vi "ThreeIncoming.vi"() -> ()   [LabVIEW 2013]
uses:
  <vilib>/rvi/Emulation/niFpgaSctlEmulationGetInTimedLoop.vi
  <vilib>/rvi/Emulation/niFpgaEmulationReportErrorSimple.vi
  <vilib>/rvi/Emulation/niFpgaGetClockAttributes.vi
  <vilib>/rvi/interface/RandomDataEmulation/nirviRandomDataFPGAFIFO.vi
  <vilib>/rvi/interface/RandomDataEmulation/niFpgaRandomDataHandleErrors.vi
  <vilib>/rvi/Emulation/niFpgaCriticalErrorInLSC.vi
  <vilib>/rvi/DataTransferAndStorage/Container/XNode/niFpgaContainer.xnode
  <vilib>/rvi/interface/RandomDataEmulation/nirviRandomDataFpgaReadWriteTemplate.vi
panel:
  out "Boolean 2":bool=TRUE
  out "Fast timeout":bool
  out "Med timeout":bool
  out "Slow timeout":bool
  in  "I16":i16
  in  "I8":i8
  in  "I64":i64
  in  "I32":i32
  in  "U16":u16
  in  "U8":u8
  in  "U64":u64
  in  "U32":u32
  in  "SGL":sgl
  in  "Boolean":bool
  out "I16 out":i16
  out "I8 out":i8
  out "I64 out":i64
  out "I32 out":i32
  out "U16 out":u16
  out "U8 out":u8
  out "U64 out":u64
  out "U32 out":u32
  out "SGL out":sgl
  out "Boolean out":bool
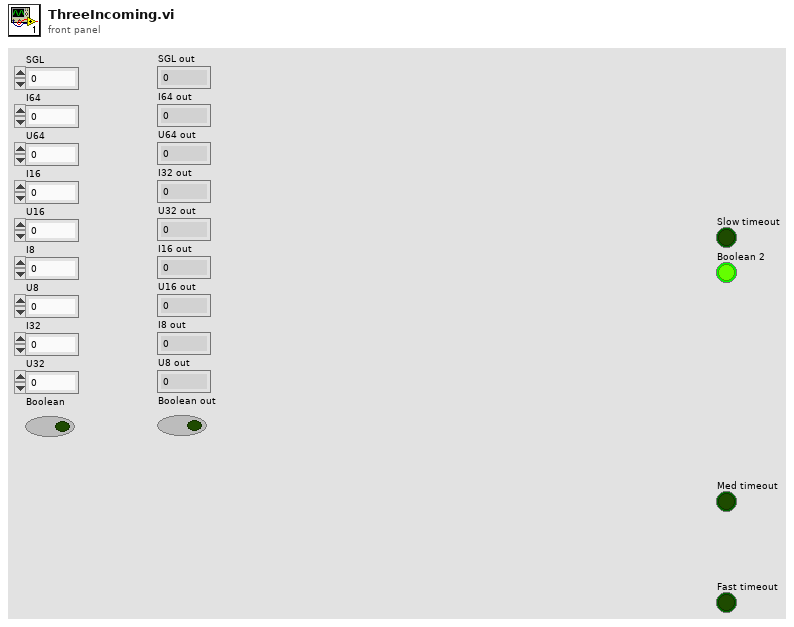
[diagram p1: front panel]
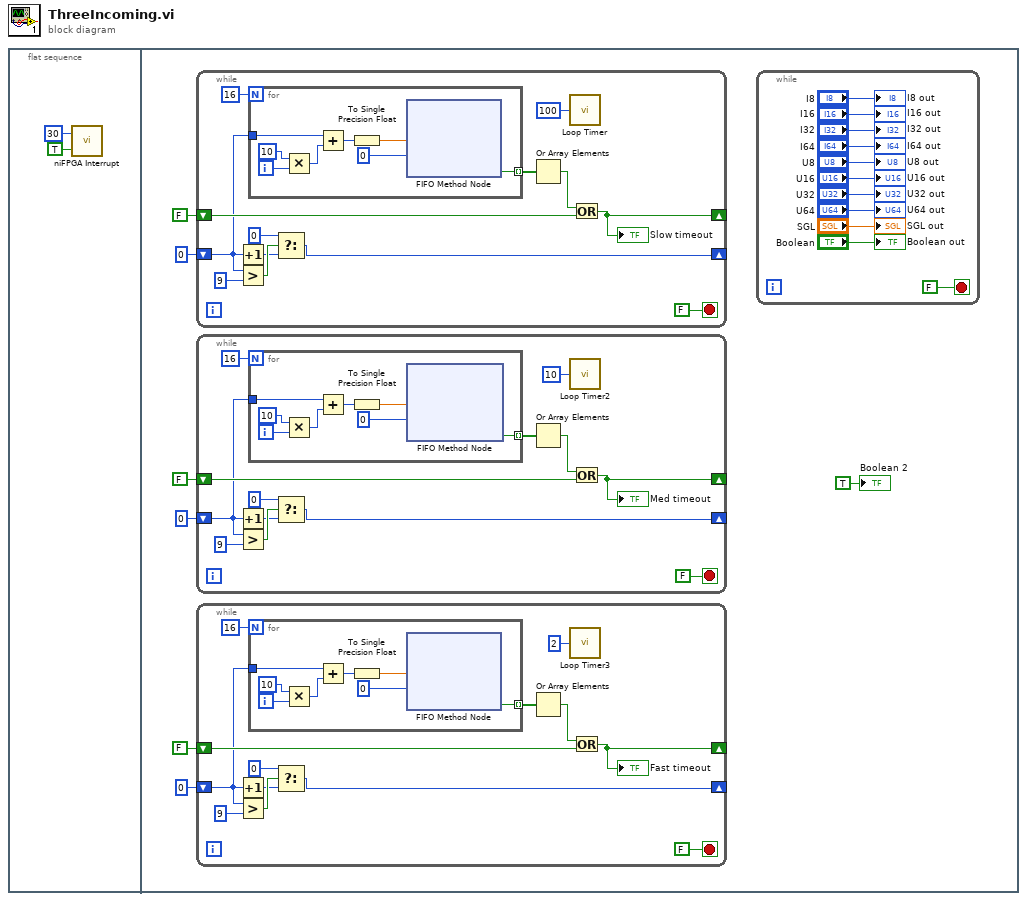
[diagram p0: block diagram]
diagram:
  n1 = flat-sequence {
    frame #0 {
      n2 = call <vilib>:"niFPGA Interrupt.vi"("Wait Until Cleared (F)"=TRUE, "IRQ Number (0)"=u8 30) -> ()  [unwired: 1 in]
    }
    frame #1 {
      n3 = while {
        shift-right: [w59] -> _
        shift-left: 0 ("t") -> [w52]
        shift-right: [w53] -> _
        shift-left: FALSE -> [w54]
        stop <- FALSE stop-if-true
        n4 = Increment(x=w52) -> (x+1=w57:i32)
        n5 = Greater?(x=w52, y=9) -> (0:w63:bool)
        n6 = for {
          N: 16 -> [_]
          tunnel: w52 -> [w72]
          tunnel: [w65] -> w56 mode=indexing
          i -> [w71]
          n7 = Multiply(x=10, y=w71) -> (x*y=w69:i32)
          n8 = Add(x=w72, y=w69) -> (x+y=w68:i32)
          n9 = To Single Precision Float(number=w68) -> (single precision float=w67:sgl)
          n10 = xnode ("FIFO Method Node")("Element"=w67, "Timeout"=0) -> ("Timed Out?"=w65:bool)  [unwired: 1 in, 1 out]
        }
        n11 = Select(t=0, s=w63, f=w57) -> (s? t:f=w59:i32)
        n12 = Or Array Elements(Boolean array=w56) -> (logical OR=w55:bool)
        n13 = call "Loop Timer"("Count(uSec)"=u32 100) -> ()  [unwired: 1 out]
        n14 = Or(x=w55, y=w54) -> (x .or. y?=w53:bool)
        "Slow timeout" <- w53
      }
      n15 = while {
        shift-right: [w38] -> _
        shift-left: 0 ("t") -> [w31]
        shift-right: [w32] -> _
        shift-left: FALSE -> [w33]
        stop <- FALSE stop-if-true
        n16 = Increment(x=w31) -> (x+1=w36:i32)
        n17 = Greater?(x=w31, y=9) -> (0:w42:bool)
        n18 = for {
          N: 16 -> [_]
          tunnel: w31 -> [w51]
          tunnel: [w44] -> w35 mode=indexing
          i -> [w50]
          n19 = Multiply(x=10, y=w50) -> (x*y=w48:i32)
          n20 = Add(x=w51, y=w48) -> (x+y=w47:i32)
          n21 = To Single Precision Float(number=w47) -> (single precision float=w46:sgl)
          n22 = xnode ("FIFO Method Node")("Element"=w46, "Timeout"=0) -> ("Timed Out?"=w44:bool)  [unwired: 1 in, 1 out]
        }
        n23 = Select(t=0, s=w42, f=w36) -> (s? t:f=w38:i32)
        n24 = Or Array Elements(Boolean array=w35) -> (logical OR=w34:bool)
        n25 = call "Loop Timer2"("Count(uSec)"=u32 10) -> ()  [unwired: 1 out]
        n26 = Or(x=w34, y=w33) -> (x .or. y?=w32:bool)
        "Med timeout" <- w32
      }
      n27 = while {
        shift-right: [w17] -> _
        shift-left: 0 ("t") -> [w10]
        shift-right: [w11] -> _
        shift-left: FALSE -> [w12]
        stop <- FALSE stop-if-true
        n28 = Increment(x=w10) -> (x+1=w15:i32)
        n29 = Greater?(x=w10, y=9) -> (0:w21:bool)
        n30 = for {
          N: 16 -> [_]
          tunnel: w10 -> [w30]
          tunnel: [w23] -> w14 mode=indexing
          i -> [w29]
          n31 = Multiply(x=10, y=w29) -> (x*y=w27:i32)
          n32 = Add(x=w30, y=w27) -> (x+y=w26:i32)
          n33 = To Single Precision Float(number=w26) -> (single precision float=w25:sgl)
          n34 = xnode ("FIFO Method Node")("Element"=w25, "Timeout"=0) -> ("Timed Out?"=w23:bool)  [unwired: 1 in, 1 out]
        }
        n35 = Select(t=0, s=w21, f=w15) -> (s? t:f=w17:i32)
        n36 = Or Array Elements(Boolean array=w14) -> (logical OR=w13:bool)
        n37 = call "Loop Timer3"("Count(uSec)"=u32 2) -> ()  [unwired: 1 out]
        n38 = Or(x=w13, y=w12) -> (x .or. y?=w11:bool)
        "Fast timeout" <- w11
      }
      n39 = while {
        stop <- FALSE stop-if-true
        "I16 out" <- "I16"
        "I8 out" <- "I8"
        "I64 out" <- "I64"
        "I32 out" <- "I32"
        "U16 out" <- "U16"
        "U8 out" <- "U8"
        "U64 out" <- "U64"
        "U32 out" <- "U32"
        "SGL out" <- "SGL"
        "Boolean out" <- "Boolean"
      }
      "Boolean 2" <- TRUE
    }
  }
